vi "Periodic Tasks.vi"(8 "error in":errorcluster) -> ()   [LabVIEW 2017]
doc: "This VI runs in parallel to other tasks. It can contain as many user-defined periodic loops as you need. These can carry out PID or other sorts of timed response."
uses:
  _SHARE ALL/RoboRio Share All/Systems Share All/Joystick/Joystick.lvlib
  _SHARE ALL/RoboRio Share All/Systems Share All/System_Monitoring/System_Status.lvlib
  Systems/SRXSubSystem/SRX SubSystem.lvlib
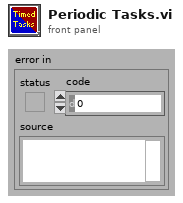
[diagram p1: front panel]
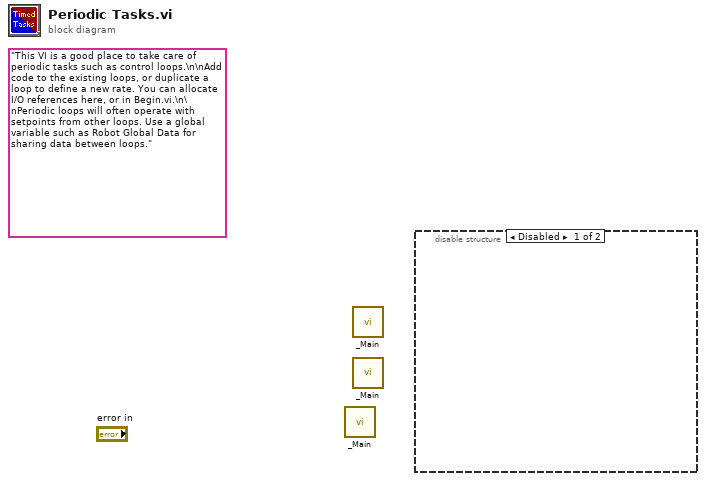
[diagram p0: block diagram]
diagram:
  (unwired) "This VI is a good place to take care of periodic tasks such as control loops.\n\nAdd code to the existing loops, or duplicate a loop to define a new rate. You can allocate I/O references here, or in Begin.vi.\n\nPeriodic loops will often operate with setpoints from other loops. Use a global variable such as Robot Global Data for sharing data between loops."
  n1 = call "_Main.vi"() -> ()  [unwired: 12 in]
  n2 = call "_Main.vi"() -> ()  [unwired: 12 in]
  n3 = call "_Main.vi"() -> ()  [unwired: 12 in]
  n4 = disable-structure shown="Disabled" {
    frame Disabled {
    }
    frame Enabled {
    }
  }
